vi "Write Scalar Data.vi"(8 "error in (no error)":errorcluster, 9 "Changed?":bool[](array[boolean]), 10 "Values":dbl[](array[numeric]), 11 "Cluster":T1={"Name"="", "Data Type"=enum."<Null>", "session"=0, "Scalar Type"=enum."Standard", "Index"=0, "Length"=0, "attributes"=variant(refnum<k20> refnum), "default value"=variant(refnum<k20> refnum)} {"Data Type" format="%.0x"}) -> (0 "error out":errorcluster, 2 "Values":dbl[](array[numeric]))   [LabVIEW 2018, in "FPGA Addon Engine.lvlib"]
uses:
  FPGA Addon Engine.lvlib
  Types/Register Settings.ctl
  Addon Shared/Types/Data Type.ctl
  Addon Shared/Types/Scalar Type.ctl
  APIs/FPGA Register IO/Write Methods/Write Data Register/Instances/Write I8.vi
  APIs/FPGA Register IO/Write Methods/Write Data Register/Instances/Write I16.vi
  APIs/FPGA Register IO/Write Methods/Write Data Register/Instances/Write I32.vi
  APIs/FPGA Register IO/Write Methods/Write Data Register/Instances/Write I64.vi
  APIs/FPGA Register IO/Write Methods/Write Data Register/Instances/Write U8.vi
  APIs/FPGA Register IO/Write Methods/Write Data Register/Instances/Write U16.vi
  APIs/FPGA Register IO/Write Methods/Write Data Register/Instances/Write U32.vi
  APIs/FPGA Register IO/Write Methods/Write Data Register/Instances/Write U64.vi
  APIs/FPGA Register IO/Write Methods/Write Data Register/Instances/Write SGL.vi
  APIs/FPGA Register IO/Write Methods/Write Data Register/Instances/Write FXP.vi
  APIs/FPGA Register IO/FPGA Register IO.lvlib
  Addon Shared/FPGA Addon Shared.lvlib
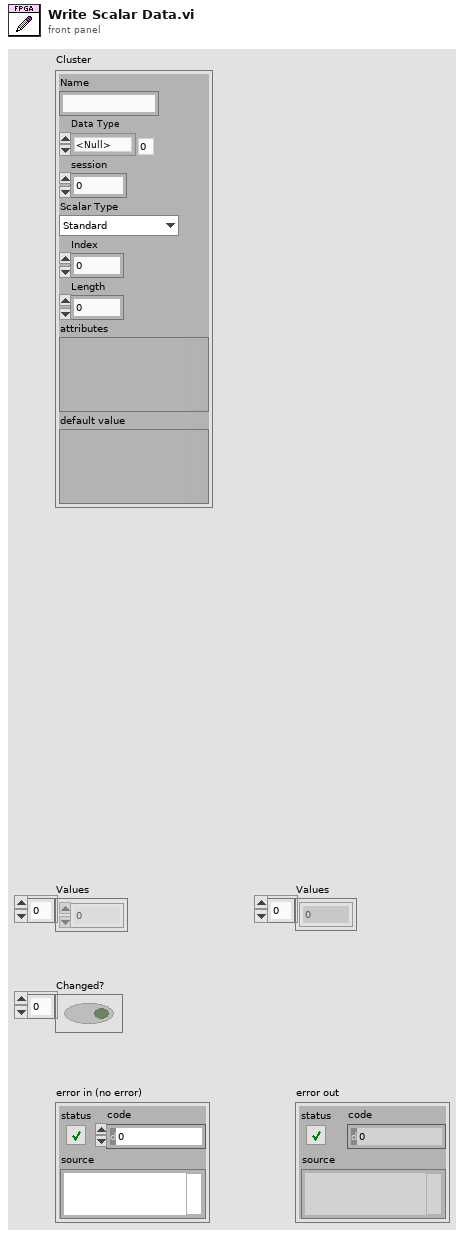
[diagram p1: front panel]
types:
  T1 = typedef "FPGA Addon Engine.lvlib/Register Settings.ctl" = cluster{"Name":string, "Data Type":T2, "session":u32, "Scalar Type":T3, "Index":i32, "Length":i32, "attributes":variant, "default value":variant}
  T2 = typedef "FPGA Addon Shared.lvlib/Data Type.ctl" = enum8{"<Null>", "I8", "I16", "I32", "I64", "U8", "U16", "U32", "U64", "SGL", "Boolean", "Analog PWM In Settings", "Analog PWM In", "Digital PWM In Settings", "Digital PWM In", "Digital PWM Out", "Sine Out", "FXP+/-24.5", "FXP+/-16.5", "FXP+/-32.8", "FXP+/-64.32", "FXP+/-16.7", "FXP+/-20.5", "FXP+/-27.5", "FXP+/-32.16", "FXP+16.3", "FXP+18.3", "Digital Static In", "Digital Static Out", "Digital Static In Settings", "Digital WSS Out", "Quad Encoder Settings", "Quad Encoder In", "Group"}
  T3 = typedef "FPGA Addon Shared.lvlib/Scalar Type.ctl" = enum16{"Standard", "Bitpacked"}
  T4 = cluster{"ACTIVE EDGE":bool, "TIMEOUT":u32, "THRESHOLD":fxp<+/-,32,8>}
  T5 = cluster{"ACTIVE EDGE":bool, "ACTIVE TICKS":u32, "INACTIVE TICKS":u32, "DATA":u8, "SENSOR TYPE":u8}
  T6 = cluster{"AMP":fxp<+/-,32,8>, "OFFSET":fxp<+/-,32,8>, "PERIODS/TICKS":fxp<+,32,0>}
  T7 = cluster{"DIRECTION":u8, "RESET VALUE":i32, "A RESET STATE":bool, "B RESET STATE":bool, "Z RESET STATE":bool}
  T8 = cluster{"ACTIVE EDGE":bool, "ACTIVE TICKS":u32, "INACTIVE TICKS":u32}
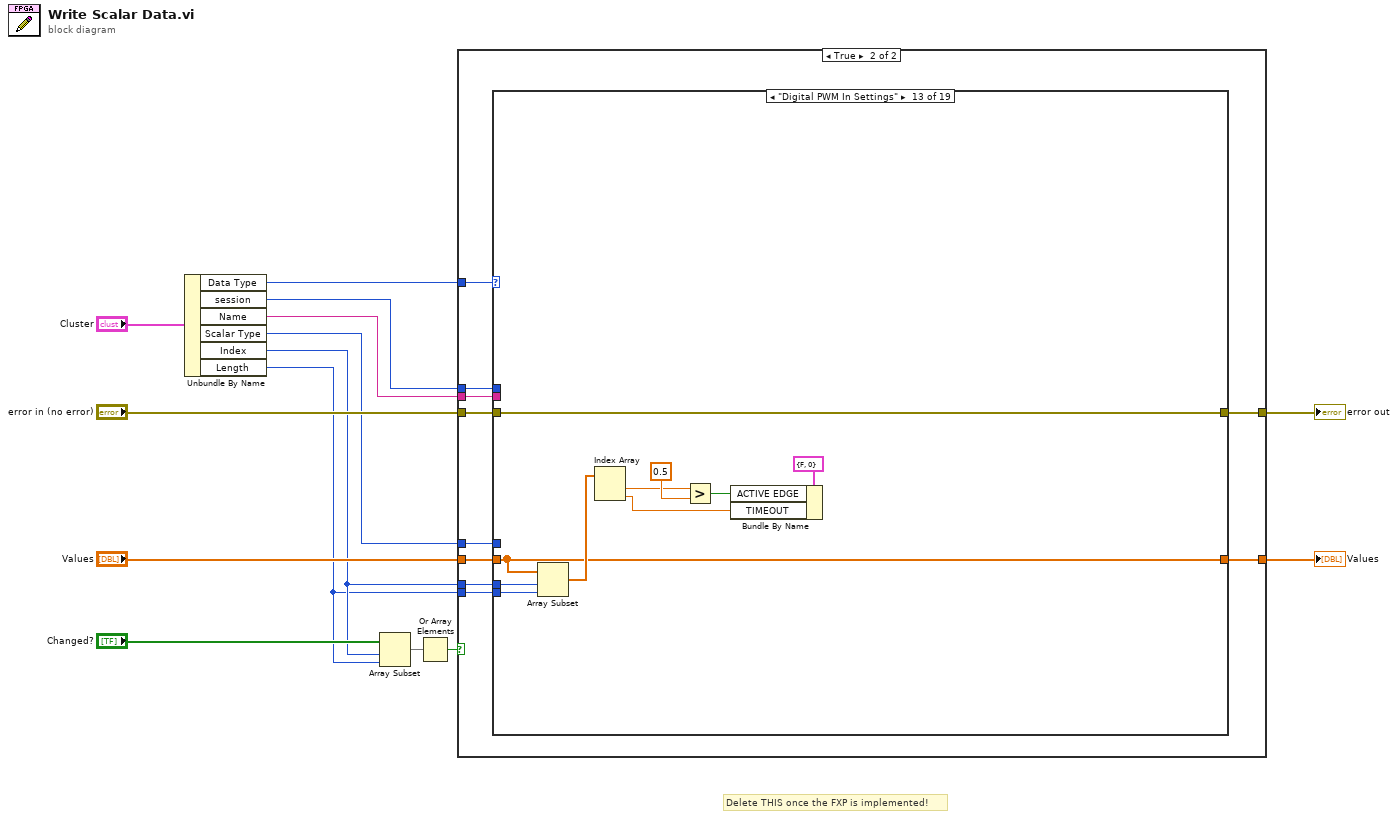
[diagram p0: block diagram]
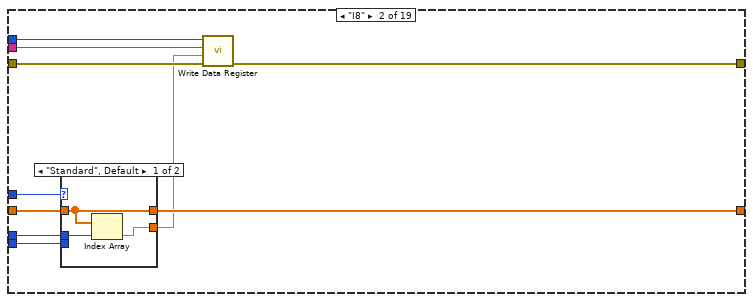
[diagram p4: hidden frame]
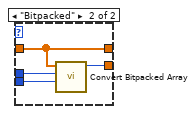
[diagram p5: hidden frame]
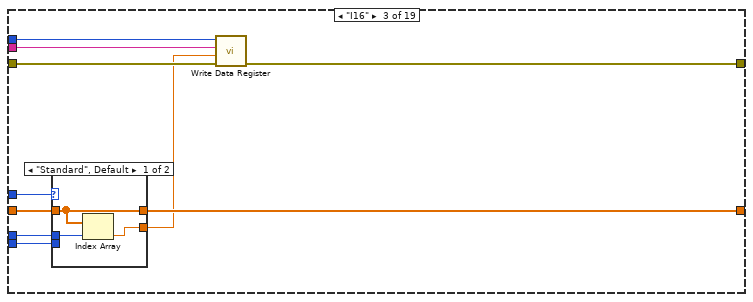
[diagram p6: hidden frame]
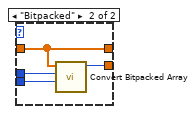
[diagram p7: hidden frame]
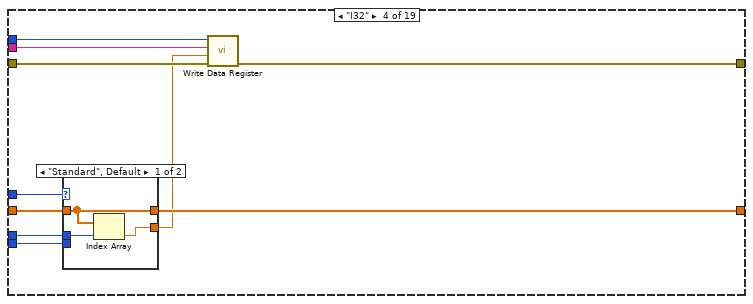
[diagram p8: hidden frame]
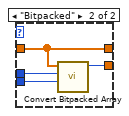
[diagram p9: hidden frame]
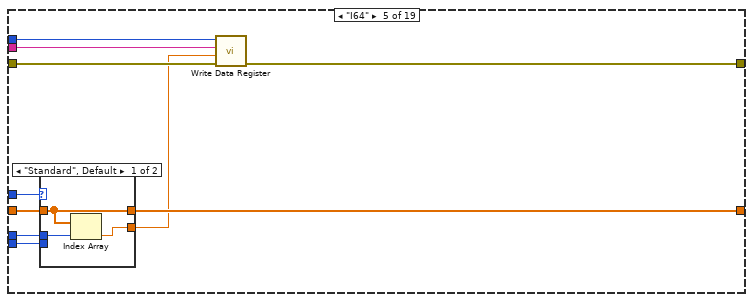
[diagram p10: hidden frame]
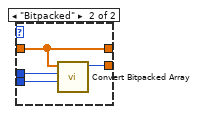
[diagram p11: hidden frame]
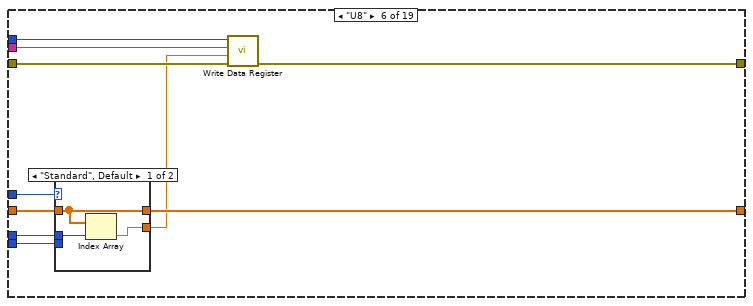
[diagram p12: hidden frame]
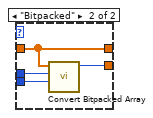
[diagram p13: hidden frame]
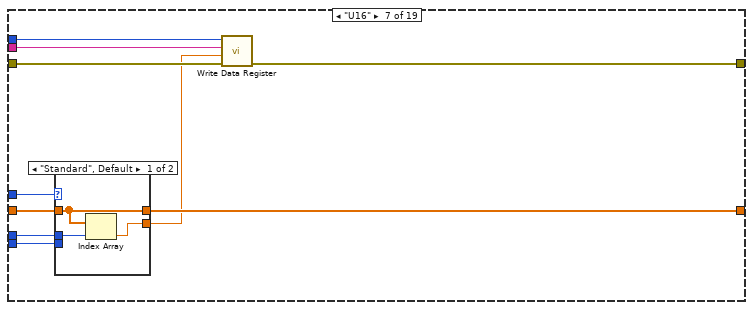
[diagram p14: hidden frame]
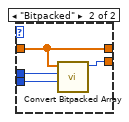
[diagram p15: hidden frame]
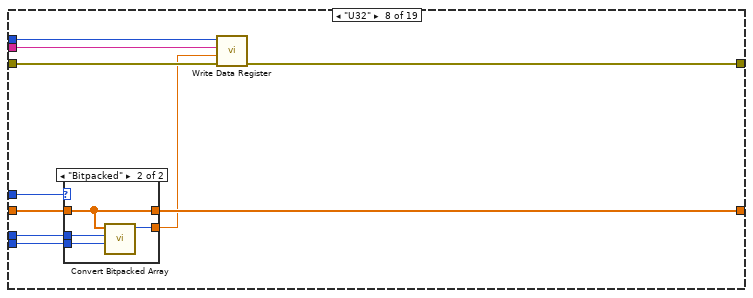
[diagram p16: hidden frame]
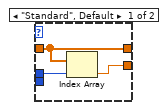
[diagram p17: hidden frame]
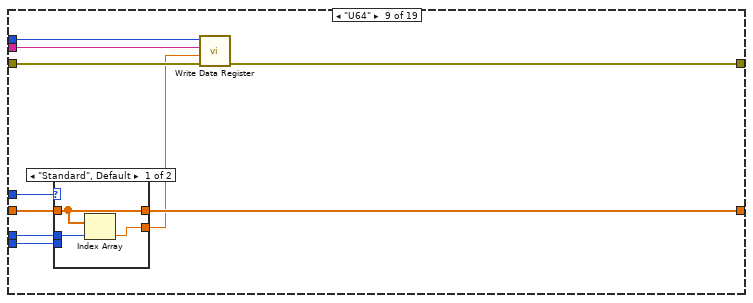
[diagram p18: hidden frame]
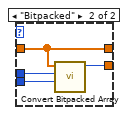
[diagram p19: hidden frame]
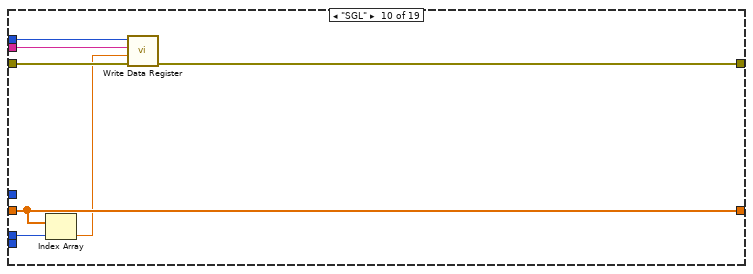
[diagram p20: hidden frame]
diagram:
  # "Delete THIS once the FXP is implemented!"
  n1 = Unbundle By Name("Cluster") -> ("Data Type"=w7:T2, "session"=w4:u32, "Name"=w5:string, "Scalar Type"=w6:T3, "Index"=w3:i32, "Length"=w2:i32)
  n2 = Array Subset(array="Changed?", index=w3, length=w2) -> (w9:bool[])
  n3 = Or Array Elements(Boolean array=w9) -> (logical OR=w8:bool)
  n4 = case shown="True" w8 {
    tunnel: "error in (no error)" -> [w16 w26]
    tunnel: [w16 w25] -> w13
    tunnel: [w15 w24] -> w12
    tunnel: "Values" -> [w15 w23]
    tunnel: w6 -> [_ w22]
    tunnel: w2 -> [_ w21]
    tunnel: w3 -> [_ w18]
    tunnel: w7 -> [_ w20]
    tunnel: w5 -> [_ w19]
    tunnel: w4 -> [_ w17]
    frame False {
    }
    frame True {
      n5 = case shown="\"Digital PWM In Settings\"" w20 {
        tunnel: w26 -> [w28 w35 w51 w67 w84 w103 w119 w136 w154 w169 w175 w181 w192 w204 w224 w235 w244 w255 w272]
        tunnel: [w28 w34 w52 w68 w86 w102 w120 w137 w153 w170 w176 w181 w192 w204 w224 w235 w244 w255 w272] -> w25
        tunnel: [w27 w36 w53 w69 w87 w104 w121 w138 w155 w171 w178 w184 w193 w202 w222 w232 w242 w253 w267] -> w24
        tunnel: w23 -> [w27 w38 w55 w72 w89 w106 w123 w140 w157 w171 w178 w184 w193 w202 w222 w232 w242 w253 w267]
        tunnel: w22 -> [_ w37 w54 w71 w88 w105 w122 w139 w156 _ _ _ _ _ _ _ _ _ _]
        tunnel: w21 -> [_ w30 w47 w70 w81 w98 w115 w132 w149 _ _ w183 w194 w203 w223 w234 w243 w254 w270]
        tunnel: w19 -> [_ w33 w50 w65 w85 w101 w118 w135 w152 w168 w174 _ _ _ _ _ _ _ _]
        tunnel: w18 -> [_ w31 w48 w64 w82 w99 w116 w133 w150 w166 w173 w180 w191 w201 w221 w233 w241 w252 w271]
        tunnel: w17 -> [_ w29 w46 w63 w80 w97 w114 w131 w148 w165 w172 _ _ _ _ _ _ _ _]
        frame "<Null>", Default {
        }
        frame "I8" {
          n6 = case shown="\"Standard\", Default" w37 {
            tunnel: w38 -> [w40 w44]
            tunnel: [w41 w45] -> w32
            tunnel: [w40 w44] -> w36
            tunnel: w31 -> [w39 w43]
            tunnel: w30 -> [_ w42]
            frame "Standard", Default {
              n7 = Index Array(array=w40, index=w39) -> (element=w41:dbl)
            }
            frame "Bitpacked" {
              n8 = call "Convert Bitpacked Array.vi"("Length"=w42, "Index"=w43, "Values"=w44) -> ("Numeric"=w45:u64)  [unwired: 8 in]
            }
          }
          n9 = call-poly "Write Data Register.vi"("error in"=w35, "value in"=w32, "register name"=w33, "session in"=w29) -> ("error out"=w34:errorcluster)  [unwired: 6 in, 1 out]
        }
        frame "I16" {
          n10 = case shown="\"Standard\", Default" w54 {
            tunnel: w55 -> [w57 w61]
            tunnel: [w58 w62] -> w49
            tunnel: [w57 w61] -> w53
            tunnel: w48 -> [w56 w60]
            tunnel: w47 -> [_ w59]
            frame "Standard", Default {
              n11 = Index Array(array=w57, index=w56) -> (element=w58:dbl)
            }
            frame "Bitpacked" {
              n12 = call "Convert Bitpacked Array.vi"("Length"=w59, "Index"=w60, "Values"=w61) -> ("Numeric"=w62:u64)  [unwired: 8 in]
            }
          }
          n13 = call-poly "Write Data Register.vi"("error in"=w51, "value in"=w49, "register name"=w50, "session in"=w46) -> ("error out"=w52:errorcluster)  [unwired: 6 in, 1 out]
        }
        frame "I32" {
          n14 = case shown="\"Standard\", Default" w71 {
            tunnel: w72 -> [w74 w78]
            tunnel: w70 -> [_ w76]
            tunnel: [w75 w79] -> w66
            tunnel: [w74 w78] -> w69
            tunnel: w64 -> [w73 w77]
            frame "Standard", Default {
              n15 = Index Array(array=w74, index=w73) -> (element=w75:dbl)
            }
            frame "Bitpacked" {
              n16 = call "Convert Bitpacked Array.vi"("Length"=w76, "Index"=w77, "Values"=w78) -> ("Numeric"=w79:u64)  [unwired: 8 in]
            }
          }
          n17 = call-poly "Write Data Register.vi"("error in"=w67, "value in"=w66, "register name"=w65, "session in"=w63) -> ("error out"=w68:errorcluster)  [unwired: 6 in, 1 out]
        }
        frame "I64" {
          n18 = case shown="\"Standard\", Default" w88 {
            tunnel: w89 -> [w91 w95]
            tunnel: [w92 w96] -> w83
            tunnel: [w91 w95] -> w87
            tunnel: w82 -> [w90 w94]
            tunnel: w81 -> [_ w93]
            frame "Standard", Default {
              n19 = Index Array(array=w91, index=w90) -> (element=w92:dbl)
            }
            frame "Bitpacked" {
              n20 = call "Convert Bitpacked Array.vi"("Length"=w93, "Index"=w94, "Values"=w95) -> ("Numeric"=w96:u64)  [unwired: 8 in]
            }
          }
          n21 = call-poly "Write Data Register.vi"("error in"=w84, "value in"=w83, "register name"=w85, "session in"=w80) -> ("error out"=w86:errorcluster)  [unwired: 6 in, 1 out]
        }
        frame "U8" {
          n22 = case shown="\"Standard\", Default" w105 {
            tunnel: w106 -> [w108 w112]
            tunnel: [w109 w113] -> w100
            tunnel: [w108 w112] -> w104
            tunnel: w99 -> [w107 w111]
            tunnel: w98 -> [_ w110]
            frame "Standard", Default {
              n23 = Index Array(array=w108, index=w107) -> (element=w109:dbl)
            }
            frame "Bitpacked" {
              n24 = call "Convert Bitpacked Array.vi"("Length"=w110, "Index"=w111, "Values"=w112) -> ("Numeric"=w113:u64)  [unwired: 8 in]
            }
          }
          n25 = call-poly "Write Data Register.vi"("error in"=w103, "value in"=w100, "register name"=w101, "session in"=w97) -> ("error out"=w102:errorcluster)  [unwired: 6 in, 1 out]
        }
        frame "U16" {
          n26 = case shown="\"Standard\", Default" w122 {
            tunnel: w123 -> [w125 w129]
            tunnel: [w126 w130] -> w117
            tunnel: [w125 w129] -> w121
            tunnel: w116 -> [w124 w128]
            tunnel: w115 -> [_ w127]
            frame "Standard", Default {
              n27 = Index Array(array=w125, index=w124) -> (element=w126:dbl)
            }
            frame "Bitpacked" {
              n28 = call "Convert Bitpacked Array.vi"("Length"=w127, "Index"=w128, "Values"=w129) -> ("Numeric"=w130:u64)  [unwired: 8 in]
            }
          }
          n29 = call-poly "Write Data Register.vi"("error in"=w119, "value in"=w117, "register name"=w118, "session in"=w114) -> ("error out"=w120:errorcluster)  [unwired: 6 in, 1 out]
        }
        frame "U32" {
          n30 = case shown="\"Bitpacked\"" w139 {
            tunnel: w140 -> [w142 w146]
            tunnel: [w143 w147] -> w134
            tunnel: [w142 w146] -> w138
            tunnel: w133 -> [w141 w145]
            tunnel: w132 -> [_ w144]
            frame "Standard", Default {
              n31 = Index Array(array=w142, index=w141) -> (element=w143:dbl)
            }
            frame "Bitpacked" {
              n32 = call "Convert Bitpacked Array.vi"("Length"=w144, "Index"=w145, "Values"=w146) -> ("Numeric"=w147:u64)  [unwired: 8 in]
            }
          }
          n33 = call-poly "Write Data Register.vi"("error in"=w136, "value in"=w134, "register name"=w135, "session in"=w131) -> ("error out"=w137:errorcluster)  [unwired: 6 in, 1 out]
        }
        frame "U64" {
          n34 = case shown="\"Standard\", Default" w156 {
            tunnel: w157 -> [w159 w163]
            tunnel: [w160 w164] -> w151
            tunnel: [w159 w163] -> w155
            tunnel: w150 -> [w158 w162]
            tunnel: w149 -> [_ w161]
            frame "Standard", Default {
              n35 = Index Array(array=w159, index=w158) -> (element=w160:dbl)
            }
            frame "Bitpacked" {
              n36 = call "Convert Bitpacked Array.vi"("Length"=w161, "Index"=w162, "Values"=w163) -> ("Numeric"=w164:u64)  [unwired: 8 in]
            }
          }
          n37 = call-poly "Write Data Register.vi"("error in"=w154, "value in"=w151, "register name"=w152, "session in"=w148) -> ("error out"=w153:errorcluster)  [unwired: 6 in, 1 out]
        }
        frame "SGL" {
          n38 = Index Array(array=w171, index=w166) -> (element=w167:dbl)
          n39 = call-poly "Write Data Register.vi"("error in"=w169, "value in"=w167, "register name"=w168, "session in"=w165) -> ("error out"=w170:errorcluster)  [unwired: 6 in, 1 out]
        }
        frame "Boolean" {
          n40 = Index Array(array=w178, index=w173) -> (element=w177:dbl)
          n41 = To Unsigned Byte Integer(number=w177) -> (unsigned 8bit integer=w179:u8)
          n42 = Greater Than 0?(x=w179) -> ()  [unwired: 1 out]
          n43 = call-poly "Write Data Register.vi"("error in"=w175, "register name"=w174, "session in"=w172) -> ("error out"=w176:errorcluster)  [unwired: 7 in, 1 out]
        }
        frame "Analog PWM In Settings" {
          n44 = Array Subset(array=w184, index=w180, length=w183) -> (w190:dbl[])
          n45 = Index Array(array=w190) -> (element #1=w188:dbl, element #2=w186:dbl, element #3=w185:dbl)  [unwired: 4 in, 1 out]
          n46 = Greater?(x=w188, y=0.5) -> (0:w187:bool)
          n47 = Bundle By Name(cluster=T4 {"ACTIVE EDGE"=FALSE, "TIMEOUT"=0, "THRESHOLD"=0.0} ("Value"), "ACTIVE EDGE"=w187, "TIMEOUT"=w186, "THRESHOLD"=w185) -> ()  [unwired: 1 out]
        }
        frame "Digital PWM In Settings" {
          n48 = Array Subset(array=w193, index=w191, length=w194) -> (w200:dbl[])
          n49 = Index Array(array=w200) -> (element #1=w197:dbl, element #2=w196:dbl)  [unwired: 2 in]
          n50 = Greater?(x=w197, y=0.5) -> (0:w199:bool)
          n51 = Bundle By Name(cluster=cluster{"ACTIVE EDGE":bool, "TIMEOUT":u32} {"ACTIVE EDGE"=FALSE, "TIMEOUT"=0} ("Value"), "ACTIVE EDGE"=w199, "TIMEOUT"=w196) -> ()  [unwired: 1 out]
        }
        frame "Digital WSS Out" {
          # "Speed\nData\nPPR\nWD\nSensor"
          n52 = Array Subset(array=w202, index=w201, length=w203) -> (w220:dbl[])
          n53 = Index Array(array=w220) -> (element #1=w218:dbl, element #2=w217:dbl, element #3=w216:dbl, element #4=w215:dbl, element #5=w214:dbl)  [unwired: 5 in]
          n54 = Absolute Value(x=w218) -> (abs(x)=w205:dbl)
          n55 = To Single Precision Float(number=w215) -> (single precision float=w209:sgl)
          n56 = To Single Precision Float(number=w205) -> (single precision float=w211:sgl)
          n57 = To Single Precision Float(number=w216) -> (single precision float=w210:sgl)
          n58 = call "WSS_Data_Conversion.vi"("WD"=w209, "PPR"=w210, "Speed"=w211) -> ("Inactive"=w207:u32, "Active"=w208:u32)  [unwired: 7 in]
          n59 = To Unsigned Byte Integer(number=w217) -> (unsigned 8bit integer=w212:u8)
          n60 = To Unsigned Byte Integer(number=w214) -> (unsigned 8bit integer=w213:u8)
          n61 = Bundle By Name(cluster=T5 {"ACTIVE EDGE"=TRUE, "ACTIVE TICKS"=0, "INACTIVE TICKS"=0, "DATA"=0, "SENSOR TYPE"=0} ("Settings"), "ACTIVE EDGE"=TRUE, "ACTIVE TICKS"=w208, "INACTIVE TICKS"=w207, "DATA"=w212, "SENSOR TYPE"=w213) -> ()  [unwired: 1 out]
        }
        frame "Sine Out" {
          n62 = Array Subset(array=w222, index=w221, length=w223) -> (w231:dbl[])
          n63 = Index Array(array=w231) -> (element #1=w227:dbl, element #2=w228:dbl, element #3=w229:dbl)  [unwired: 3 in]
          n64 = Divide(x=w229, y=sgl 40000000.0) -> (x/y=w226:dbl)
          n65 = Bundle By Name(cluster=T6 {"AMP"=0.0, "OFFSET"=0.0, "PERIODS/TICKS"=0.0} ("Value"), "AMP"=w227, "OFFSET"=w228, "PERIODS/TICKS"=w226) -> ()  [unwired: 1 out]
        }
        frame "Digital Static In Settings" {
          n66 = Array Subset(array=w232, index=w233, length=w234) -> (w237:dbl[])
          n67 = Index Array(array=w237) -> (element=w240:dbl)  [unwired: 1 in]
          n68 = Greater?(x=w240, y=0.5) -> (0:w238:bool)
          n69 = Bundle By Name(cluster=cluster{"ACTIVE EDGE":bool} {"ACTIVE EDGE"=FALSE} ("Value"), "ACTIVE EDGE"=w238) -> ()  [unwired: 1 out]
        }
        frame "Digital Static Out" {
          w248 = 0.5 ("y")
          n70 = Array Subset(array=w242, index=w241, length=w243) -> (w251:dbl[])
          n71 = Index Array(array=w251) -> (element #1=w249:dbl, element #2=w247:dbl)  [unwired: 2 in]
          n72 = Greater?(x=w249, y=w248) -> (0:w245:bool)
          n73 = Greater?(x=w247, y=w248) -> (0:w246:bool)
          n74 = Bundle By Name(cluster=cluster{"ACTIVE EDGE":bool, "OUTPUT":bool} {"ACTIVE EDGE"=FALSE, "OUTPUT"=FALSE} ("Value"), "ACTIVE EDGE"=w245, "OUTPUT"=w246) -> ()  [unwired: 1 out]
        }
        frame "Quad Encoder Settings" {
          w259 = 0.5 ("y")
          n75 = Array Subset(array=w253, index=w252, length=w254) -> (w266:dbl[])
          n76 = Index Array(array=w266) -> (element #1=w256:dbl, element #2=w257:dbl, element #3=w260:dbl, element #4=w261:dbl, element #5=w262:dbl)  [unwired: 5 in]
          n77 = Greater?(x=w260, y=w259) -> (0:w258:bool)
          n78 = Greater?(x=w261, y=w259) -> (0:w264:bool)
          n79 = Greater?(x=w262, y=w259) -> (0:w265:bool)
          n80 = Bundle By Name(cluster=T7 {"DIRECTION"=0, "RESET VALUE"=0, "A RESET STATE"=FALSE, "B RESET STATE"=FALSE, "Z RESET STATE"=FALSE} ("Value"), "DIRECTION"=w256, "RESET VALUE"=w257, "A RESET STATE"=w258, "B RESET STATE"=w264, "Z RESET STATE"=w265) -> ()  [unwired: 1 out]
        }
        frame "Digital PWM Out" {
          n81 = Array Subset(array=w267, index=w271, length=w270) -> (w289:dbl[])
          n82 = Index Array(array=w289) -> (element #1=w286:dbl, element #2=w284:dbl, element #3=w285:dbl)  [unwired: 3 in]
          n83 = To Single Precision Float(number=w285) -> (single precision float=w277:sgl)
          n84 = To Single Precision Float(number=w284) -> (single precision float=w278:sgl)
          n85 = In Range and Coerce(upper limit=sgl 100.0, x=w277, lower limit=sgl 0.0) -> (coerced(x)=w276:sgl)  [unwired: 1 out]
          n86 = Equal To 0?(x=w278) -> (x = 0?=w283:bool)
          n87 = Divide(x=sgl 40000000.0 ("y"), y=w278) -> (x/y=w281:sgl)
          n88 = Multiply(x=w276, y=sgl 0.01 ("x")) -> (x*y=w279:sgl)
          n89 = case shown="True" w283 {
            tunnel: [w294 w295] -> w282
            tunnel: w281 -> [w294 _]
            tunnel: [w293 w295] -> w280
            tunnel: w279 -> [w293 _]
            frame False {
            }
            frame True {
              w295 = sgl 0.0
            }
          }
          n90 = Greater?(x=w286, y=0.5) -> (0:w287:bool)
          n91 = To Unsigned Long Integer(number=w282) -> (unsigned 32bit integer=w291:u32)
          n92 = Multiply(x=w282, y=w280) -> (x*y=w268:u32)
          n93 = Subtract(x=w291, y=w268) -> (x-y=w269:u32)
          n94 = Bundle By Name(cluster=T8 {"ACTIVE EDGE"=FALSE, "ACTIVE TICKS"=0, "INACTIVE TICKS"=0} ("Value"), "ACTIVE EDGE"=w287, "INACTIVE TICKS"=w269, "ACTIVE TICKS"=w268) -> ()  [unwired: 1 out]
        }
      }
    }
  }
  "error out" <- w13
  "Values" <- w12
